vi "GUI_Tapedrive_ESP301.vi"() -> ()   [LabVIEW 2013]
uses:
  Device Driver/shared/OnOffTypeDef.ctl
  Device Driver/Tapedrive_ESP301/Tapedrive_VIs_CK/Direction.ctl
panel:
  in  "shotnumber":i32
  out "indecator ref array":refnum<vi>[](array[refnum])
  in  "time to wait (TCP) 2":i32=10
  in  "plot":bool=TRUE
  out "ratio(h)":bool
  out "fixsize":bool
  out "error (h)":bool
  out "Device Name (h)":string="StagingDG645 1"
  in  "Main Tap":T1(tab)
  in  "Tab Control":enum32{"Move", "Tension"}(tab)
  in  "MoveDecceleration.Axis 2":dbl
  in  "MoveDecceleration.Axis 1":dbl
  in  "MoveAcceleration.Axis 2":dbl
  in  "MoveAcceleration.Axis 1":dbl
  in  "MoveVelocity.Axis 2":dbl
  in  "MoveVelocity.Axis 1":dbl
  in  "Timeout":u32
  in  "Stepsize":dbl
  in  "Direction":T2
  in  "MoveIfScan":T3 caption="Move if\nin Scanmode"
  in  "TensionDecceleration.Axis 2":dbl
  in  "TensionDecceleration.Axis 1":dbl
  in  "TensionAcceleration.Axis 2":dbl
  in  "TensionAcceleration.Axis 1":dbl
  in  "TensionVelocity.Axis 2":dbl
  in  "TensionVelocity.Axis 1":dbl
  in  "Tension":T3
  in  "TapeRelax":dbl
  in  "Power.Axis 2":T3
  in  "Power.Axis 1":T3
  in  "Velocity.Axis 2":dbl
  in  "Velocity.Axis 1":dbl
  in  "Decceleration.Axis 2":dbl
  in  "Decceleration.Axis 1":dbl
  in  "Acceleration.Axis 2":dbl
  in  "Acceleration.Axis 1":dbl
  in  "tapepos":dbl
  in  "HomeEncoder":T3
  in  "GoStep":T3
  out "status":T4(ring) caption="Status"
  in  "Abort":bool=TRUE
  out "inmotion":T3
  out "local Port":u16=65427
  out "port or service name":u16=65426
  out "Remote Host":string="192.168.11.97"
  in  "timeout ms (slow resp)":i32=500
  in  "reset":bool
  out "image con closed":bool
  out "image \nconnection":bool
  out "image con closed 2":bool=TRUE
  out "All Devices (h)":string[](array[string])=["StagingDG645 1", "StagingDG645 2"]
  in  "time to wait (TCP)":i32=10
  out "error out":errorcluster
  out "connections (hidden)":variant[](array[variant])=[variant(refnum<k16> refnum), variant(refnum<k16> refnum)]
  in  "time to wait (main loop)":i32=10
  out "Data String":string="Amplitude.Ch AB,3.000000000000\r\nAmplitude.Ch CD,4.000000000000\r\nAmplitude.Ch EF,4.000000000000\r\nAmplitude.Ch GH,4.000000000000\r\nAmplitude.Ch T0,4.000000000000\r\nDelay.Ch A,0.000000000000\r\nDelay.Ch B,0.030000000000\r\nDelay.Ch C,0.000000000000\r\nDelay.Ch D,0.030000000000\r\nDelay.Ch E,0.000000000000\r\nDelay.Ch F,0.030000000000\r\nDelay.Ch G,0.000000000000\r\nDelay.Ch H,0.030000000000\r\nDelay.Ch T0,0.000000000000\r\nDelay.Ch T1,0.030000\r\nInhibit,Triggers\r\nLinked.Ch A,T0\r\nLinked.Ch B,A\r\nLinked.Ch C,T0\r\nLinked.Ch D,C\r\nLinked.Ch E,T0\r\nLinked.Ch F,E\r\nLinked.Ch G,T0\r\nLinked.Ch H,G\r\nLocalSavingPath,c:\\temp\r\nSave,off\r\nTrigger.ExecuteSingleShot,\r\nTrigger.Level,1.000000\r\nTrigger.Rate,10.000000\r\nTrigger.Source,External rising edges\r\ntimeout,0.000000\r\nPolarity.Ch AB,Positive\r\nPolarity.Ch CD,Positive\r\nPolarity.Ch EF,Positive\r\nPolarity.Ch GH,Positive\r\nPolarity.Ch T0,Positive\r\n"
  in  "Local Saving Path":path
  in  "MaxStepsize":dbl
  in  "get Values":bool=TRUE
  in  "MaxVelocity.Axis 1":dbl
  in  "MaxAcceleration.Axis 1":dbl
  in  "MaxAcceleration.Axis 2":dbl
  in  "VelocityFFG.Axis 1":dbl
  in  "VelocityFFG.Axis 2":dbl
  in  "AccelerationFFG.Axis 1":dbl
  in  "AccelerationFFG.Axis 2":dbl
  in  "DACoffset.Axis 1":dbl
  in  "DACoffset.Axis 2":dbl
  in  "MaxVelocity.Axis 2":dbl
  in  "StopWait":T3
  out "error message":string
  # "Move Parameters"
  # "FORWARD"
  # "BACKWARD"
  # "Tension Parameters"
  # "FORWARD"
  # "BACKWARD"
  # "Actual Axis Parameters"
  # "FORWARD"
  # "BACKWARD"
  # "Advanced Axis Parameters"
  # "AXIS  1 = forward"
  # "AXIS  2 = backward"
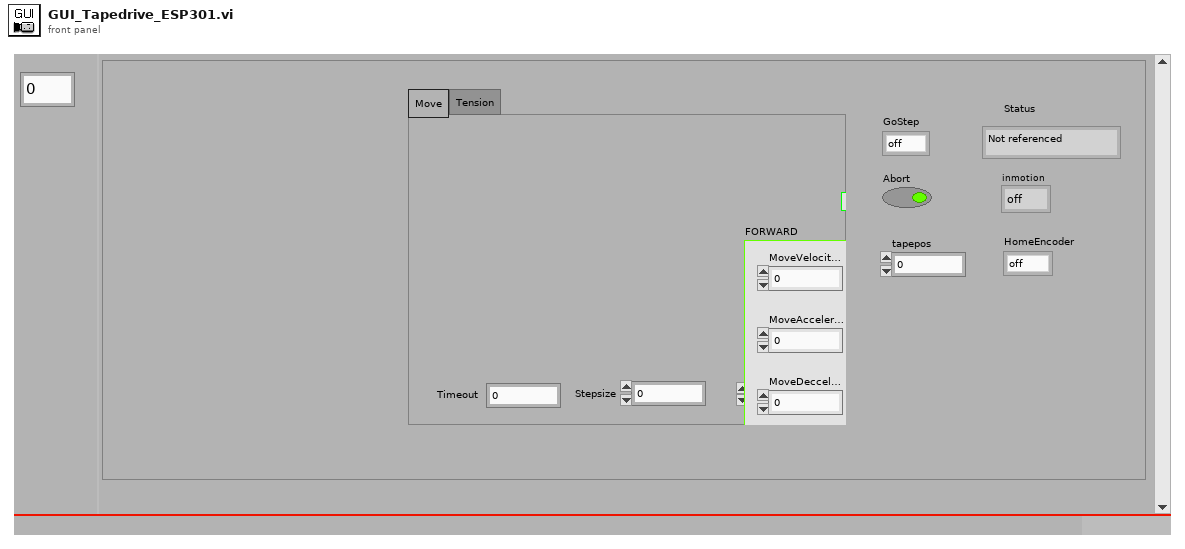
[diagram p1: front panel]
types:
  T1 = enum32{"All Channels", "Network", "Internal", "Advanced"}
  T2 = typedef "Direction.ctl" = enum16{"Forward", "Backward", "Undefined"}
  T3 = typedef "OnOffTypeDef.ctl" = enum16{"off", "on"}
  T4 = enum16{"Not referenced", "Homing", "Moving", "Ready"}
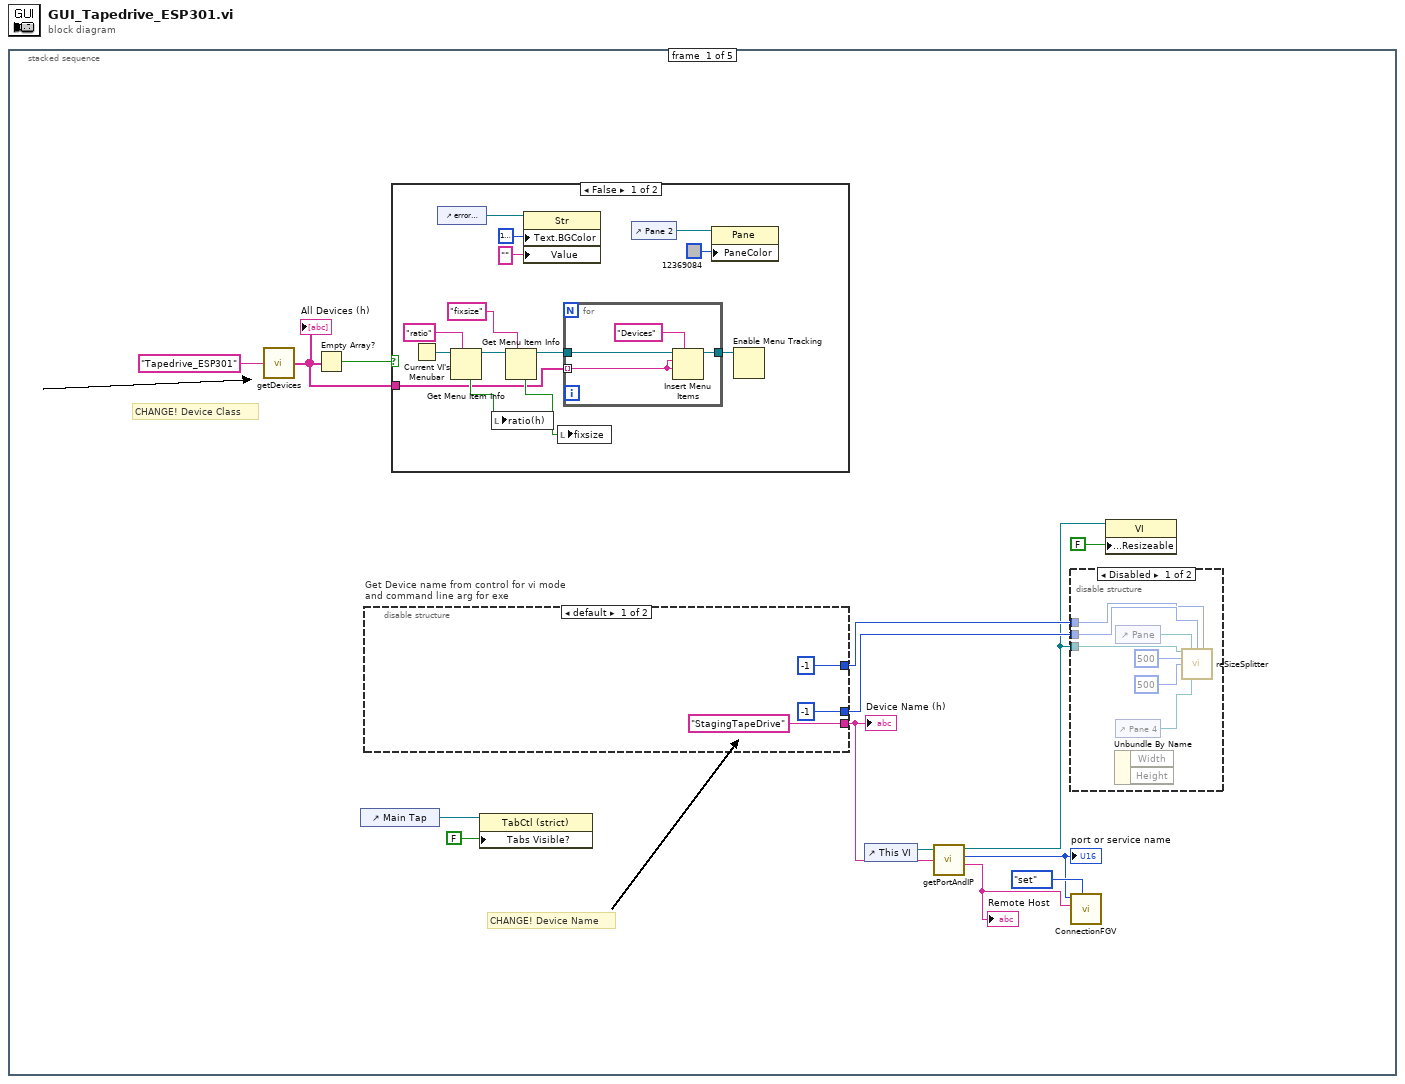
[diagram p0: block diagram]
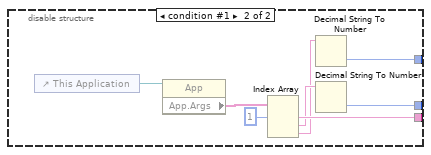
[diagram p4: hidden frame]
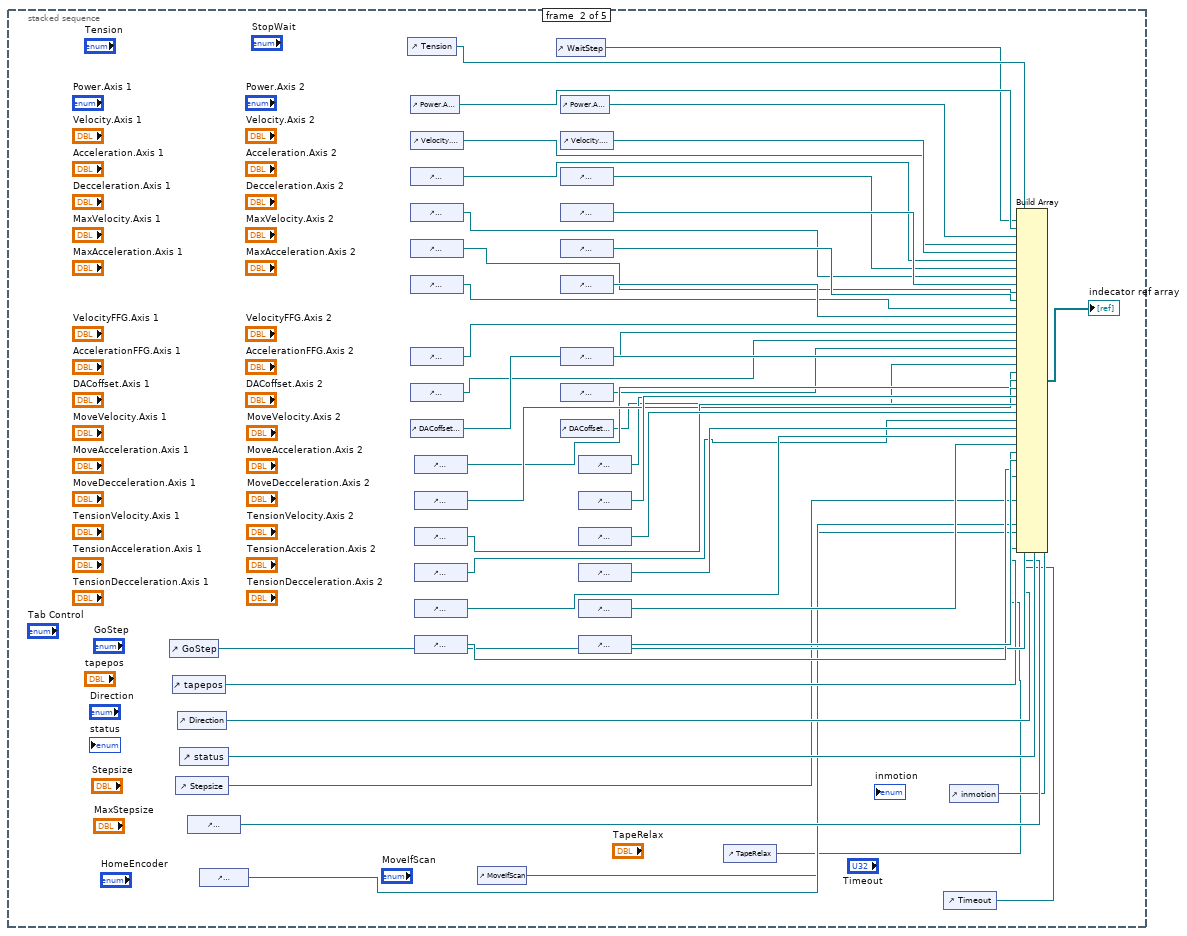
[diagram p5: hidden frame]
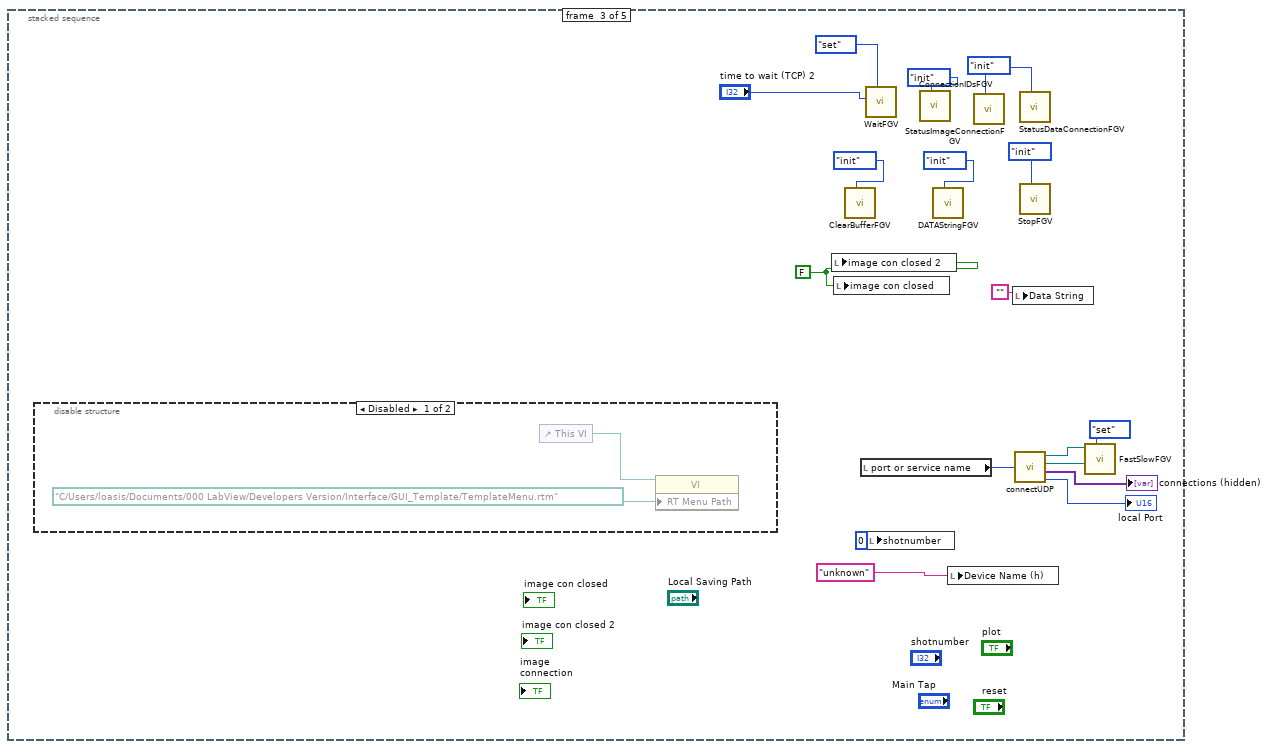
[diagram p6: hidden frame]
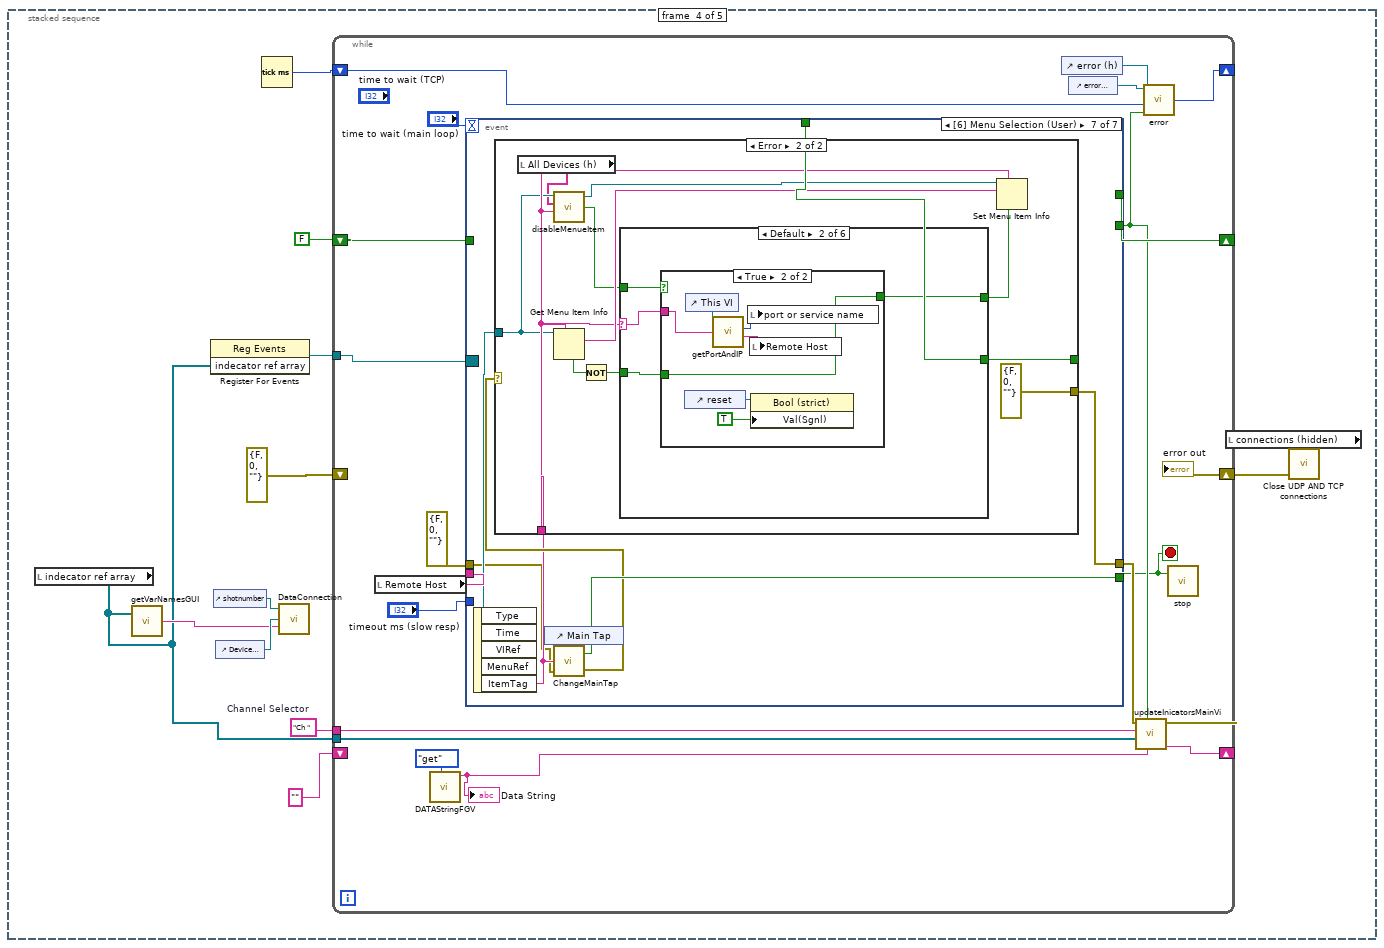
[diagram p8: hidden frame]
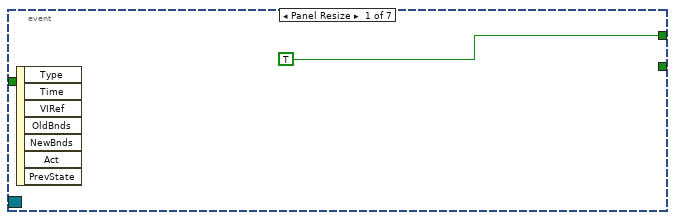
[diagram p9: hidden frame]
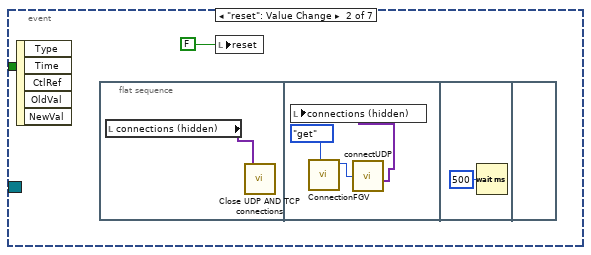
[diagram p10: hidden frame]
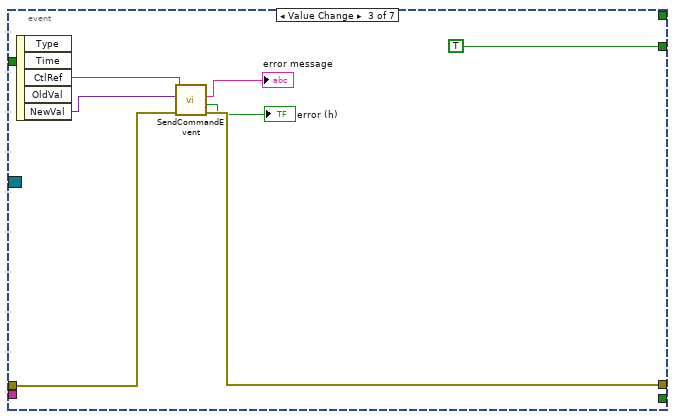
[diagram p11: hidden frame]
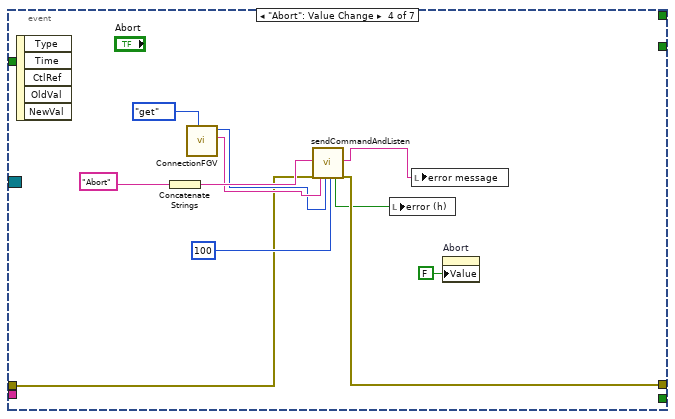
[diagram p12: hidden frame]
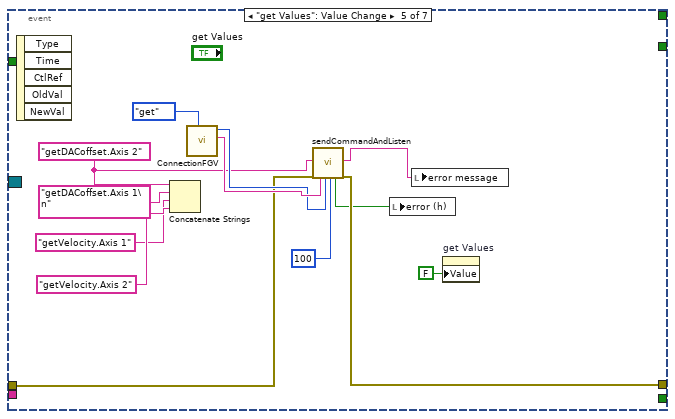
[diagram p13: hidden frame]
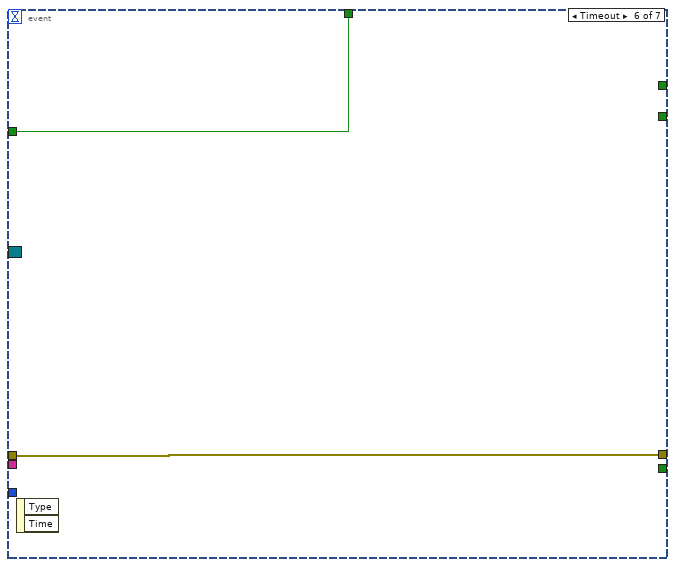
[diagram p14: hidden frame]
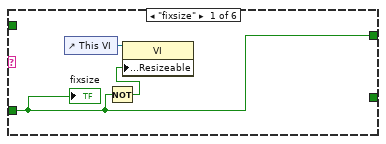
[diagram p16: hidden frame]
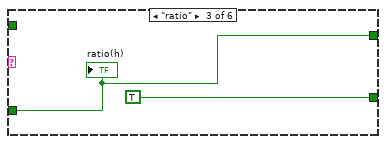
[diagram p18: hidden frame]
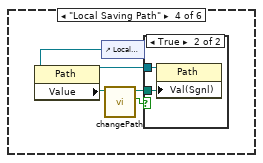
[diagram p19: hidden frame]
diagram:
  n1 = stacked-sequence {
    frame #0 {
      # "CHANGE! Device Name"
      # "CHANGE! Device Class"
      n2 = call "getDevices.vi"("Device Class"="Tapedrive_ESP301") -> ("All Devices"=w1:string[])
      "All Devices (h)" <- w1
      n3 = Empty Array?(array=w1) -> (empty?=w2:bool)
      n4 = control-ref of="Main Tap"() -> (w14:refnum<vi>)
      n5 = disable-structure "Get Device name from control for vi mode\nand command line arg for exe" shown="default" {
        disable-tunnel: ["StagingTapeDrive" ("Device Name for vi mode") w47] -> w10
        disable-tunnel: [i16 -1 ("left") w44] -> w12
        disable-tunnel: [i16 -1 ("left") w43] -> w11
        frame condition #0 (active) {
        }
        frame condition #1 {
          n6 = control-ref of="This Application"() -> (w50:refnum<vi>)
          n7 = property class="App"(reference=w50) -> ("App.Args"=w49:string[])  [unwired: 1 in, 2 out]
          n8 = Index Array(array=w49, index #1=1 ("index")) -> (element #1=w47:string, element #2=w46:string, element #3=w45:string)  [unwired: 2 in]
          n9 = Decimal String To Number(string=w45) -> (number=w43:i32)  [unwired: 2 in, 1 out]
          n10 = Decimal String To Number(string=w46) -> (number=w44:i32)  [unwired: 2 in, 1 out]
        }
      }
      "Device Name (h)" <- w10
      n11 = case shown="False" w2 {
        tunnel: w1 -> [w15 _]
        frame False {
          n12 = Current VI's Menubar() -> (w27:refnum<k9>)
          n13 = control-ref of="error message"() -> (w21:refnum<vi>)
          n14 = Get Menu Item Info(7:"ratio" ("item tag"), 11:w27) -> (3:w25:refnum<k9>, 4:w26:bool)  [unwired: 1 in, 5 out]
          n15 = local write "ratio(h)"(w26) -> ()
          n16 = Get Menu Item Info(7:"fixsize" ("item tag"), 11:w25) -> (3:w17:refnum<k9>, 4:w23:bool)  [unwired: 1 in, 5 out]
          n17 = property class="Str"(reference=w21, "Text.BGColor"=u32 16777238, "Value"="") -> ()  [unwired: 1 in, 2 out]
          n18 = local write "fixsize"(w23) -> ()
          n19 = for {
            tunnel: w17 -> [w32]
            tunnel: [w31] -> w16
            tunnel: w15 -> [w29] mode=indexing
            n20 = Insert Menu Items(5:"Devices" ("menu tag"), 7:w29, 8:w29, 9:w32) -> (3:w31:refnum<k9>)  [unwired: 2 in, 2 out]
          }
          n21 = control-ref of="Pane 2"() -> (w19:refnum<vi>)
          n22 = property class="Pane"(reference=w19, "PaneColor"=u32 12369084) -> ()  [unwired: 1 in, 2 out]
          n23 = Enable Menu Tracking(4:w16) -> ()  [unwired: 2 in, 2 out]
        }
        frame True {
        }
      }
      n24 = property class="TabCtl (strict)"(reference=w14, "Tabs Visible?"=FALSE) -> ()  [unwired: 1 in, 2 out]
      n25 = control-ref of="This VI"() -> (w9:refnum<vi>)
      n26 = call "getPortAndIP.vi"("Device Name"=w10, "This Vi"=w9) -> ("Remote Host"=w5:string, "port or service name"=w4:u16, "reference out"=w7:refnum<vi>)  [unwired: 2 in, 2 out]
      "port or service name" <- w4
      "Remote Host" <- w5
      n27 = disable-structure shown="Disabled" {
        disable-tunnel: w12 -> [w38 _]
        disable-tunnel: w11 -> [w37 _]
        disable-tunnel: w7 -> [w35 _]
        frame Disabled {
          n28 = Unbundle By Name() -> ()  [unwired: 1 in, 2 out]
          n29 = control-ref of="Pane"() -> (w39:refnum<vi>)
          n30 = control-ref of="Pane 4"() -> (w36:refnum<vi>)
          n31 = call "reSizeSplitter.vi"("this vi"=w35, "pane"=w39, "left"=w38, "top"=w37, "Width"=u32 500, "Height"=u32 500, "pane2"=w36) -> ()  [unwired: 8 in, 1 out]
        }
        frame Enabled {
        }
      }
      n32 = call "ConnectionFGV.vi"("command"=enum16{"get", "set", "init"}."set", "Remote Host in"=w5, "port or service name in"=w4) -> ()  [unwired: 7 in, 2 out]
      n33 = property class="VI"(reference=w7, "Front Panel.Resizeable"=FALSE ("Front Panel Window:Resizable")) -> ()  [unwired: 1 in, 2 out]
    }
    frame #1 {
      n34 = control-ref of="GoStep"() -> (w63:refnum<vi>)
      n35 = control-ref of="tapepos"() -> (w62:refnum<vi>)
      n36 = control-ref of="Stepsize"() -> (w59:refnum<vi>)
      n37 = control-ref of="Direction"() -> (w61:refnum<vi>)
      n38 = control-ref of="status"() -> (w60:refnum<vi>)
      n39 = control-ref of="MaxStepsize"() -> (w58:refnum<vi>)
      n40 = control-ref of="HomeEncoder"() -> (w54:refnum<vi>)
      n41 = control-ref of="Tension"() -> (w56:refnum<vi>)
      n42 = control-ref of="Power.Axis 1"() -> (w65:refnum<vi>)
      n43 = control-ref of="Velocity.Axis 1"() -> (w67:refnum<vi>)
      n44 = control-ref of="Acceleration.Axis 1"() -> (w69:refnum<vi>)
      n45 = control-ref of="Decceleration.Axis 1"() -> (w71:refnum<vi>)
      n46 = control-ref of="MaxVelocity.Axis 1"() -> (w73:refnum<vi>)
      n47 = control-ref of="MaxAcceleration.Axis 1"() -> (w75:refnum<vi>)
      n48 = control-ref of="VelocityFFG.Axis 1"() -> (w77:refnum<vi>)
      n49 = control-ref of="AccelerationFFG.Axis 1"() -> (w79:refnum<vi>)
      n50 = control-ref of="DACoffset.Axis 1"() -> (w81:refnum<vi>)
      n51 = control-ref of="MoveVelocity.Axis 1"() -> (w83:refnum<vi>)
      n52 = control-ref of="MoveAcceleration.Axis 1"() -> (w85:refnum<vi>)
      n53 = control-ref of="MoveDecceleration.Axis 1"() -> (w87:refnum<vi>)
      n54 = control-ref of="TensionVelocity.Axis 1"() -> (w89:refnum<vi>)
      n55 = control-ref of="TensionAcceleration.Axis 1"() -> (w91:refnum<vi>)
      n56 = control-ref of="TensionDecceleration.Axis 1"() -> (w93:refnum<vi>)
      n57 = control-ref of="MoveIfScan"() -> (w53:refnum<vi>)
      n58 = control-ref of="WaitStep"() -> (w55:refnum<vi>)
      n59 = control-ref of="Power.Axis 2"() -> (w66:refnum<vi>)
      n60 = control-ref of="Velocity.Axis 2"() -> (w68:refnum<vi>)
      n61 = control-ref of="Acceleration.Axis 2"() -> (w70:refnum<vi>)
      n62 = control-ref of="Decceleration.Axis 2"() -> (w72:refnum<vi>)
      n63 = control-ref of="MaxVelocity.Axis 2"() -> (w74:refnum<vi>)
      n64 = control-ref of="MaxAcceleration.Axis 2"() -> (w76:refnum<vi>)
      n65 = control-ref of="VelocityFFG.Axis 2"() -> (w78:refnum<vi>)
      n66 = control-ref of="AccelerationFFG.Axis 2"() -> (w80:refnum<vi>)
      n67 = control-ref of="DACoffset.Axis 2"() -> (w82:refnum<vi>)
      n68 = control-ref of="MoveVelocity.Axis 2"() -> (w84:refnum<vi>)
      n69 = control-ref of="MoveAcceleration.Axis 2"() -> (w86:refnum<vi>)
      n70 = control-ref of="MoveDecceleration.Axis 2"() -> (w88:refnum<vi>)
      n71 = control-ref of="TensionVelocity.Axis 2"() -> (w90:refnum<vi>)
      n72 = control-ref of="TensionAcceleration.Axis 2"() -> (w92:refnum<vi>)
      n73 = control-ref of="TensionDecceleration.Axis 2"() -> (w94:refnum<vi>)
      n74 = control-ref of="TapeRelax"() -> (w51:refnum<vi>)
      n75 = control-ref of="Timeout"() -> (w52:refnum<vi>)
      n76 = control-ref of="inmotion"() -> (w57:refnum<vi>)
      n77 = Build Array(w56, w55, w65, w66, w67, w68, w69, w70, w71, w72, w73, w74, w75, w76, w77, w78, w79, w80, w81, w82, w83, w84, w85, w86, w87, w88, w89, w90, w91, w92, w93, w94, w63, w62, w61, w60, w59, w58, w57, w54, w53, w52, w51) -> (→"indecator ref array":refnum<vi>[])
    }
    frame #2 {
      w103 = enum16{"get", "set", "init"}."init" ("Command")
      w109 = FALSE ("new Device Data")
      n78 = disable-structure shown="Disabled" {
        frame Disabled {
          n79 = control-ref of="This VI"() -> (w113:refnum<vi>)
          n80 = property class="VI"(reference=w113, "RT Menu Path"=path "C:/Users/loasis/Documents/000 LabView/Developers Version/Interface/GUI_Template/TemplateMenu.rtm" ("Run-Time Menu Path")) -> ()  [unwired: 1 in, 2 out]
        }
        frame Enabled {
        }
      }
      n81 = local write "image con closed 2"(w109) -> ()
      n82 = local write "image con closed"(w109) -> ()
      n83 = call "ClearBufferFGV.vi"("Command"=enum16{"set", "get", "init"}."init") -> ()  [unwired: 10 in, 1 out]
      n84 = local read "port or service name"() -> (w99:u16)
      n85 = call "WaitFGV.vi"("Command"=enum16{"get", "set", "init"}."set", "milliseconds to wait"="time to wait (TCP) 2") -> ()  [unwired: 9 in, 1 out]
      n86 = local write "shotnumber"(0 ("shotnumber")) -> ()
      n87 = call "ConnectionIDsFGV.vi"("Command"=enum16{"add", "get", "init"}."init") -> ()  [unwired: 10 in, 1 out]
      n88 = call "DATAStringFGV.vi"("Command"=enum16{"get", "set", "init"}."init") -> ()  [unwired: 9 in, 2 out]
      n89 = local write "Device Name (h)"("unknown" ("Device Name")) -> ()
      n90 = call "StatusImageConnectionFGV.vi"("Command"=w103) -> ()  [unwired: 10 in, 1 out]
      n91 = local write "Data String"("") -> ()
      n92 = call "connectUDP.vi"("port or service name NOT USED"=w99) -> ("fast ID (h)"=w98:refnum<k16>, "slow ID (h)"=w97:refnum<k16>, "connections (hidden)"=→"connections (hidden)":variant[], "local Port"=→"local Port":u16)
      n93 = call "StatusDataConnectionFGV.vi"("Command"=w103) -> ()  [unwired: 10 in, 1 out]
      n94 = call "StopFGV.vi"("Command"=enum16{"set", "get", "init"}."init") -> ()  [unwired: 9 in, 2 out]
      n95 = call "FastSlowFGV.vi"("Command"=enum16{"get", "set", "init"}."set", "slow ID"=w97, "fast ID"=w98) -> ()  [unwired: 7 in, 2 out]
    }
    frame #3 {
      w116 = "Ch "  # Channel Selector
      n96 = local read "indecator ref array"() -> (w114:refnum<vi>[])
      n97 = call "getVarNamesGUI.vi"("Array"=w114) -> ("String"=w115:string)  [unwired: 1 in]
      n98 = register-events(w114) -> (reference out=w117:refnum<event-registration>)  [unwired: 2 in, 1 out]
      n99 = control-ref of="shotnumber"() -> (w119:refnum<vi>)
      n100 = control-ref of="Device Name (h)"() -> (w118:refnum<vi>)
      n101 = Tick Count (ms)() -> (millisecond timer value=w121:u32)
      n102 = call "DataConnection.vi"("Subscriber list"=w115, "Device Name (h)"=w118, "shotnumber"=w119) -> ()
      n103 = while {
        shift-right: [w141] -> w124
        shift-left: errorcluster {"status"=FALSE, "code"=0, "source"=""} ("error out") -> [_]
        tunnel: w114 -> [w135]
        shift-right: [w139] -> _
        shift-left: FALSE -> [w140]
        shift-right: [w138] -> _
        shift-left: w121 -> [w137]
        shift-right: [w128] -> _
        shift-left: "" ("Data String") -> [_]
        tunnel: w117 -> [w131]
        tunnel: w116 -> [w130]
        stop <- w132 stop-if-true
        n104 = local read "Remote Host"() -> (w143:string)
        n105 = call "DATAStringFGV.vi"("Command"=enum16{"get", "set", "init"}."get") -> ("Data String out"=w133:string)  [unwired: 9 in, 1 out]
        "Data String" <- w133
        n106 = event shown="[6] Menu Selection (User)" {
          selector: w131 -> [_ _ _ _ _ _ _]
          dyn-events: _ -> [_ _ _ _ _ _ _]
          timeout: "time to wait (main loop)" -> [_ _ _ _ _ _ _]
          tunnel: [_ _ w157 w163 w178 w185 w187] -> w142
          tunnel: w143 -> [_ _ _ _ _ _ _]
          tunnel: "timeout ms (slow resp)" -> [_ _ _ _ _ _ _]
          tunnel: errorcluster {"status"=FALSE, "code"=0, "source"=""} ("error out") -> [_ _ w154 w164 w179 w185 w188]
          tunnel: [_ _ TRUE _ _ _ _] -> w136
          tunnel: [_ _ _ _ _ _ w193] -> w132
          tunnel: [_ _ _ _ _ w184 w190] -> _
          tunnel: w140 -> [_ _ _ _ _ w184 _]
          tunnel: [TRUE _ _ _ _ _ _] -> w139
          event Panel Resize {
            n107 = event-data() -> ()  [unwired: 1 in, 7 out]
          }
          event "reset": Value Change {
            n108 = event-data() -> ()  [unwired: 1 in, 5 out]
            n109 = flat-sequence {
              frame #0 {
                n110 = local read "connections (hidden)"() -> (w148:variant[])
                n111 = call "Close UDP AND TCP connections.vi"("appended array"=w148) -> ()  [unwired: 7 in]
              }
              frame #1 {
                n112 = call "ConnectionFGV.vi"("command"=enum16{"get", "set", "init"}."get") -> ("port or service name out"=w150:u16)  [unwired: 9 in, 1 out]
                n113 = call "connectUDP.vi"("port or service name NOT USED"=w150) -> ("connections (hidden)"=w149:variant[])  [unwired: 3 out]
                n114 = local write "connections (hidden)"(w149) -> ()
              }
              frame #2 {
                n115 = Wait (ms)(milliseconds to wait=u32 500) -> ()  [unwired: 1 out]
              }
              frame #3 {
              }
            }
            n116 = local write "reset"(FALSE ("reset")) -> ()
          }
          event Value Change {
            n117 = event-data() -> ("CtlRef"=w159:refnum<vi>, "NewVal"=w158:variant)  [unwired: 1 in, 3 out]
            n118 = call "SendCommandEvent.vi"("error out 2"=w154, "NewVal"=w158, "CtlRef"=w159) -> ("error out"=w157:errorcluster, "error (h)"=→"error (h)":bool, "error message"=→"error message":string)  [unwired: 5 in, 1 out]
          }
          event "Abort": Value Change {
            n119 = event-data() -> ()  [unwired: 1 in, 5 out]
            n120 = Concatenate Strings("Abort") -> (w169:string)
            n121 = call "ConnectionFGV.vi"("command"=enum16{"get", "set", "init"}."get") -> ("Remote Host out"=w167:string, "port or service name out"=w166:u16)  [unwired: 9 in]
            n122 = call "sendCommandAndListen.vi"("command in"=w169, "error in"=w164, "Remote Host"=w167, "port or service name"=w166, "timeout ms (100)"=100) -> ("error"=w162:bool, "error message"=w161:string, "error out"=w163:errorcluster)  [unwired: 7 in, 5 out]
            n123 = local write "error (h)"(w162) -> ()
            n124 = local write "error message"(w161) -> ()
            n125 = property on="Abort" class="Bool (strict)"("Value"=FALSE ("Abort")) -> ()  [unwired: 2 in, 2 out]
          }
          event "get Values": Value Change {
            w171 = "getDACoffset.Axis 2"
            n126 = event-data() -> ()  [unwired: 1 in, 5 out]
            n127 = Concatenate Strings(w171, "getDACoffset.Axis 1\n", "getVelocity.Axis 1", "getVelocity.Axis 2") -> ()  [unwired: 1 out]
            n128 = call "ConnectionFGV.vi"("command"=enum16{"get", "set", "init"}."get") -> ("Remote Host out"=w182:string, "port or service name out"=w181:u16)  [unwired: 9 in]
            n129 = call "sendCommandAndListen.vi"("command in"=w171, "error in"=w179, "Remote Host"=w182, "port or service name"=w181, "timeout ms (100)"=100) -> ("error"=w177:bool, "error message"=w176:string, "error out"=w178:errorcluster)  [unwired: 7 in, 5 out]
            n130 = local write "error (h)"(w177) -> ()
            n131 = local write "error message"(w176) -> ()
            n132 = property on="get Values" class="Bool (strict)"("Value"=FALSE ("Abort")) -> ()  [unwired: 2 in, 2 out]
          }
          event Timeout {
            n133 = event-data() -> ()  [unwired: 1 in, 2 out]
          }
          event Menu Selection (User) {
            n134 = event-data() -> ("MenuRef"=w189:refnum<k9>, "ItemTag"=w191:string)  [unwired: 1 in, 3 out]
            n135 = control-ref of="Main Tap"() -> (w186:refnum<vi>)
            n136 = call "ChangeMainTap.vi"("error in"=w188, "ItemTag"=w191, "reference"=w186) -> ("error out"=w192:errorcluster, "Boolean"=w193:bool)
            n137 = case shown="Error" w192 {
              selector: w192 -> [w194 _]
              tunnel: w189 -> [_ w200]
              tunnel: [_ w202] -> w190
              tunnel: w191 -> [_ w201]
              tunnel: [w194 errorcluster {"status"=FALSE, "code"=0, "source"=""} ("error IO")] -> w187
              frame No Error {
              }
              frame Error {
                n138 = local read "All Devices (h)"() -> (w195:string[])
                n139 = call "disableMenueItem.vi"("ItemTag"=w201, "All Devices (h)"=w195, "MenuRef"=w200) -> ("this is a Device(tag)"=w199:bool, "menu reference out"=w198:refnum<k9>)  [unwired: 1 in, 1 out]
                n140 = Get Menu Item Info(7:w201, 11:w200) -> (2:w204:string, 4:w205:bool)  [unwired: 1 in, 5 out]
                n141 = Not(x=w205) -> (.not. x?=w203:bool)
                n142 = case shown="Default" w201 {
                  selector: w201 -> [_ w211 _ _ _ _]
                  tunnel: w203 -> [w206 w209 w220 _ _ _]
                  tunnel: [_ _ TRUE _ _ _] -> w202
                  tunnel: w199 -> [_ w212 _ _ _ _]
                  tunnel: [w206 w210 w220 _ _ _] -> w197
                  frame "fixsize" {
                    n143 = control-ref of="This VI"() -> (w208:refnum<vi>)
                    n144 = Not(x=w206) -> (.not. x?=w207:bool)
                    n145 = property class="VI"(reference=w208, "Front Panel.Resizeable"=w207) -> ()  [unwired: 1 in, 2 out]
                    "fixsize" <- w206
                  }
                  frame Default {
                    n146 = case shown="True" w212 {
                      tunnel: w211 -> [_ w219]
                      tunnel: [_ w213] -> w210
                      tunnel: w209 -> [_ w213]
                      frame False {
                      }
                      frame True {
                        n147 = control-ref of="reset"() -> (w215:refnum<vi>)
                        n148 = control-ref of="This VI"() -> (w218:refnum<vi>)
                        n149 = call "getPortAndIP.vi"("Device Name"=w219, "This Vi"=w218) -> ("Remote Host"=w217:string, "port or service name"=w216:u16)  [unwired: 2 in, 3 out]
                        n150 = local write "port or service name"(w216) -> ()
                        n151 = local write "Remote Host"(w217) -> ()
                        n152 = property class="Bool (strict)"(reference=w215, "Val(Sgnl)"=TRUE ("Value (Signaling)")) -> ()  [unwired: 1 in, 2 out]
                      }
                    }
                  }
                  frame "ratio" {
                    "ratio(h)" <- w220
                  }
                  frame "Local Saving Path" {
                    n153 = control-ref of="Local Saving Path"() -> (w222:refnum<vi>)
                    n154 = property class="Path"(reference=w222) -> (reference out=w225:refnum<vi>, "Value"=w226:path)  [unwired: 1 in, 1 out]
                    n155 = call "changePath.vi"("Local Saving in (h)"=w226) -> ("change (h)"=w224:bool, "Local Saving out (h)"=w223:path)  [unwired: 9 in]
                    n156 = case shown="True" w224 {
                      tunnel: w225 -> [_ w228]
                      tunnel: w223 -> [_ w227]
                      frame False {
                      }
                      frame True {
                        n157 = property class="Path"(reference=w228, "Val(Sgnl)"=w227) -> ()  [unwired: 1 in, 2 out]
                      }
                    }
                  }
                  frame "reset" {
                    n158 = control-ref of="reset"() -> (w230:refnum<vi>)
                    n159 = property class="Bool (strict)"(reference=w230, "Val(Sgnl)"=TRUE ("Value (Signaling)")) -> ()  [unwired: 1 in, 2 out]
                  }
                  frame "clear" {
                    n160 = control-ref of="reset"() -> (w232:refnum<vi>)
                    n161 = property class="Bool (strict)"(reference=w232, "Val(Sgnl)"=TRUE ("Value (Signaling)")) -> ()  [unwired: 1 in, 2 out]
                  }
                }
                n162 = Set Menu Item Info(6:w197, 7:w201, 10:w204, 11:w198) -> ()  [unwired: 3 in, 2 out]
              }
            }
          }
        }
        n163 = control-ref of="error (h)"() -> (w126:refnum<vi>)
        n164 = control-ref of="error message"() -> (w127:refnum<vi>)
        n165 = call "updateInicatorsMainVi.vi"("Data String out"=w133, "Boolean"=w136, "Array"=w135, "Channel Selector"=w130, "error in"=w142) -> ("Data String out 2"=w128:string, "error out"=w141:errorcluster)  [unwired: 5 in]
        "error out" <- w141
        n166 = call "error.vi"("Boolean"=w136, "millisecond timer value"=w137, "reference"=w126, "error message"=w127) -> ("millisecond timer value 2"=w138:u32)
        n167 = call "stop.vi"("Boolean"=w132) -> ()
      }
      n168 = local read "connections (hidden)"() -> (w123:variant[])
      n169 = call "Close UDP AND TCP connections.vi"("error in"=w124, "appended array"=w123) -> ()  [unwired: 6 in]
    }
    frame #4 {
      n170 = control-ref of="Main  Control"() -> (w234:refnum<vi>)
      n171 = property class="TabCtl (strict)"(reference=w234, "Tabs Visible?"=TRUE) -> ()  [unwired: 1 in, 2 out]
      n172 = property class="TabCtl (strict)"(reference=w234, "Tab Location"=enum32{"Top", "Bottom", "Left", "Right"}."Bottom") -> ()  [unwired: 1 in, 2 out]
      n173 = flat-sequence {
        frame #0 {
          n174 = Wait (ms)(milliseconds to wait=u32 0) -> ()  [unwired: 1 out]
        }
        frame #1 {
        }
        frame #2 {
          n175 = control-ref of="This VI"() -> (w239:refnum<vi>)
          n176 = case shown="True" FALSE {
            tunnel: w239 -> [w240 w243]
            tunnel: [w240 w241] -> w238
            frame False {
            }
            frame True {
              n177 = property class="VI" props=["Front Panel.Open"](reference=w243) -> (reference out=w242:refnum<vi>)  [unwired: 1 in, 2 out]
              n178 = invoke class="VI" method="FP.Close"(reference=w242) -> (reference out=w241:refnum<vi>)  [unwired: 2 in, 2 out]
            }
          }
          n179 = Close Reference(reference=w238) -> ()  [unwired: 1 in, 1 out]
        }
      }
    }
  }
